vi "Compute Gated Phase Lifetime Plot.vi"(8 "Error In":errorcluster, 9 "Compute Delta Tau":bool, 10 "Phasor Parameters":T1={"Display Parameters"={"# Points"=0, "Ramp Type"=enum."Linear", "Type of Series"=enum."1-Exp Decays", "Min tau"=0.0, "Max tau"=0.0, "Include 0"=FALSE, "Include Infinity"=FALSE}, "Phasor Parameters"={"Harmonic Frequency"=0.0, "Use f* = 1/D Frequency"=FALSE, "Calibrated Phasor"=FALSE, "Calibration Lifetime"=1e-09, "Phasor Calculation"=enum."Direct Sum", "SEPL Type"=enum."UC", "# Gates"=1.0, "Square Gate Width"=1e-09, "Show Ticks"=FALSE}, "Decay & IRF Parameters"={"Lifetime"=0.0, "IRF Offset"=0.0, "IRF Period"=0.0, "Normalized Decays"=FALSE, "IRF Model"=enum."Dirac", "IRF Parameter 1"=0.0}, "Gate Parameters"={"First Gate Start"=0.0, "Use Gate Center"=FALSE, "Gate Width"=0.0, "Gate Step"=0.0, "# Gates"=0.0, "Gate Type"=enum."Square", "Edge Width"=0.0, "Top Slope"=0.0, "Reversed Sawtooth?"=FALSE, "Analytical Computation"=FALSE, "Integration"=enum."Item 0", "Tolerance"=1.0, "# Steps"=1.0, "Type of User-defined Function"=enum."Gate", "Use Gate Step"=FALSE}, "Detector Parameters"={"Frames/Image"=0, "Gates/Frame"=0, "Bits/Frame"=0, "Multiplicity"=0, "Incident Signal"=0.0, "Poisson Signal"=FALSE}} {"Detector Parameters"."Frames/Image" min=1; "Detector Parameters"."Multiplicity" min=0; "Detector Parameters"."Bits/Frame" min=1; "Detector Parameters"."Gates/Frame" min=1; "Gate Parameters"."# Steps" min=0.0; "Gate Parameters"."Tolerance" min=0.0; "Gate Parameters"."Top Slope" min=0.0; "Gate Parameters"."Edge Width" min=0.0; "Gate Parameters"."Gate Step" min=0.0; "Gate Parameters"."# Gates" min=0.0 step=1.0; "Gate Parameters"."Gate Width" min=0.0; "Decay & IRF Parameters"."Lifetime" min=0.0; "Decay & IRF Parameters"."IRF Period" min=0.0; "Phasor Parameters"."Square Gate Width" min=0.0; "Phasor Parameters"."# Gates" min=0.0; "Phasor Parameters"."Calibration Lifetime" min=0.0; "Phasor Parameters"."Harmonic Frequency" min=0.0; "Display Parameters"."Min tau" min=0.0; "Display Parameters"."Max tau" min=0.0; "Display Parameters"."# Points" min=1 step=1}, 11 "P-tau_ph(tau) Graph Refnum":refnum<vi>) -> (0 "Error Out":errorcluster)   [LabVIEW 2019]
uses:
  SEPL Parameters.ctl
  Phasor Explorer Display Parameters.ctl
  Type of Series.ctl
  Phasor Explorer Phasor Parameters.ctl
  Phasor Calculation Type.ctl
  SEPL Type.ctl
  Phasor Explorer Decay Parameters.ctl
  IRF Model.ctl
  Phasor Explorer Gate Parameters.ctl
  Gate Type.ctl
  Type of User-defined Function.ctl
  Phasor Explorer Detector Parameters.ctl
  Phasor L_N[W] Parameters.ctl
  Phasor_Abort Parallel Computation.vi
  <vilib>/Utility/error.llb/Error Cluster From Error Code.vi
  <vilib>/ErrorRing/Error Ring.xnode
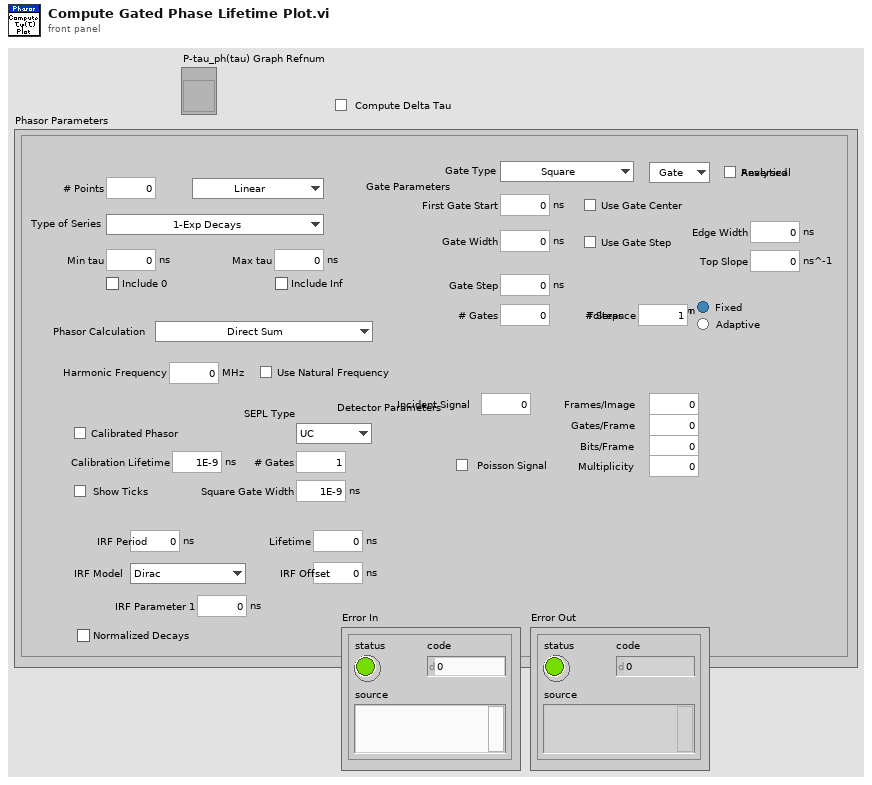
[diagram p1: front panel]
types:
  T1 = typedef "SEPL Parameters.ctl" = cluster{"Display Parameters":T2, "Phasor Parameters":T4, "Decay & IRF Parameters":T7, "Gate Parameters":T9, "Detector Parameters":T12}
  T2 = typedef "Phasor Explorer Display Parameters.ctl" = cluster{"# Points":i32, "Ramp Type":enum16{"Linear", "Logarithmic"}, "Type of Series":T3, "Min tau":dbl[unit], "Max tau":dbl[unit], "Include 0":bool, "Include Infinity":bool}
  T3 = typedef "Type of Series.ctl" = enum16{"1-Exp Decays", "Linear Combination of 1-Exp"}
  T4 = typedef "Phasor Explorer Phasor Parameters.ctl" = cluster{"Harmonic Frequency":dbl[unit], "Use f* = 1/D Frequency":bool, "Calibrated Phasor":bool, "Calibration Lifetime":dbl[unit], "Phasor Calculation":T5, "SEPL Type":T6, "# Gates":dbl, "Square Gate Width":dbl[unit], "Show Ticks":bool}
  T5 = typedef "Phasor Calculation Type.ctl" = enum16{"Direct Sum", "Analytical Formula"}
  T6 = typedef "SEPL Type.ctl" = enum16{"UC", "L_N", "L_N[W]", "L_X"}
  T7 = typedef "Phasor Explorer Decay Parameters.ctl" = cluster{"Lifetime":dbl[unit], "IRF Offset":dbl[unit], "IRF Period":dbl[unit], "Normalized Decays":bool, "IRF Model":T8, "IRF Parameter 1":dbl[unit]}
  T8 = typedef "IRF Model.ctl" = enum16{"Dirac", "Exponential"}
  T9 = typedef "Phasor Explorer Gate Parameters.ctl" = cluster{"First Gate Start":dbl[unit], "Use Gate Center":bool, "Gate Width":dbl[unit], "Gate Step":dbl[unit], "# Gates":dbl, "Gate Type":T10, "Edge Width":dbl[unit], "Top Slope":dbl[unit], "Reversed Sawtooth?":bool, "Analytical Computation":bool, "Integration":enum32{"Item 0", "Item 1"}, "Tolerance":dbl, "# Steps":dbl, "Type of User-defined Function":T11, "Use Gate Step":bool}
  T10 = typedef "Gate Type.ctl" = enum16{"Square", "Finite Edge Square", "Finite Edge, Tilted Top Square", "Triangle", "Sawtooth", "User-defined"}
  T11 = typedef "Type of User-defined Function.ctl" = enum16{"Gate", "IRF"}
  T12 = typedef "Phasor Explorer Detector Parameters.ctl" = cluster{"Frames/Image":i32, "Gates/Frame":i32, "Bits/Frame":i32, "Multiplicity":i32, "Incident Signal":dbl, "Poisson Signal":bool}
  T13 = typedef "Phasor L_N[W] Parameters.ctl" = cluster{"Laser Period":dbl[unit], "Gate Width":dbl[unit], "Gate Step":dbl[unit], "Harmonic frequency":dbl[unit], "IRF offset":dbl[unit], "# Gates":dbl}
  T14 = typedef "Gate Definitions.ctl" = cluster{"First Gate: t1":ext, "Gate Width: W":ext, "Gate Step: d":ext, "# Gates: G":ext, "Use Gate Center":bool, "Frames/Image: F":i32, "Gates/Frame: L":i32, "Bits/Frame: q":i32, "Multiplicity: p":i32, "Gate Type":T10, "Gate Edge s":ext, "Gate Top Slope":ext, "Reversed Sawtooth?":bool, "Computation":bool, "User-defined Gate":T15, "Tolerance":ext, "Integration":enum32{"Item 0", "Item 1"}, "# Steps":ext, "Type of User-defined Function":enum32{"Gate", "IRF"}}
  T15 = typedef "XY Plot Data.ctl" = cluster{"X Array":dbl[], "Y Array":dbl[]}
  T16 = typedef "Decay Definiton.ctl" = cluster{"offset: t0":ext, "period: T":ext, "lifetime: tau":ext, "Incident Signal: I":ext, "Normalized Decays":bool, "IRF Model":T8, "IRF Parameter 1":ext, "Poisson Signal":bool}
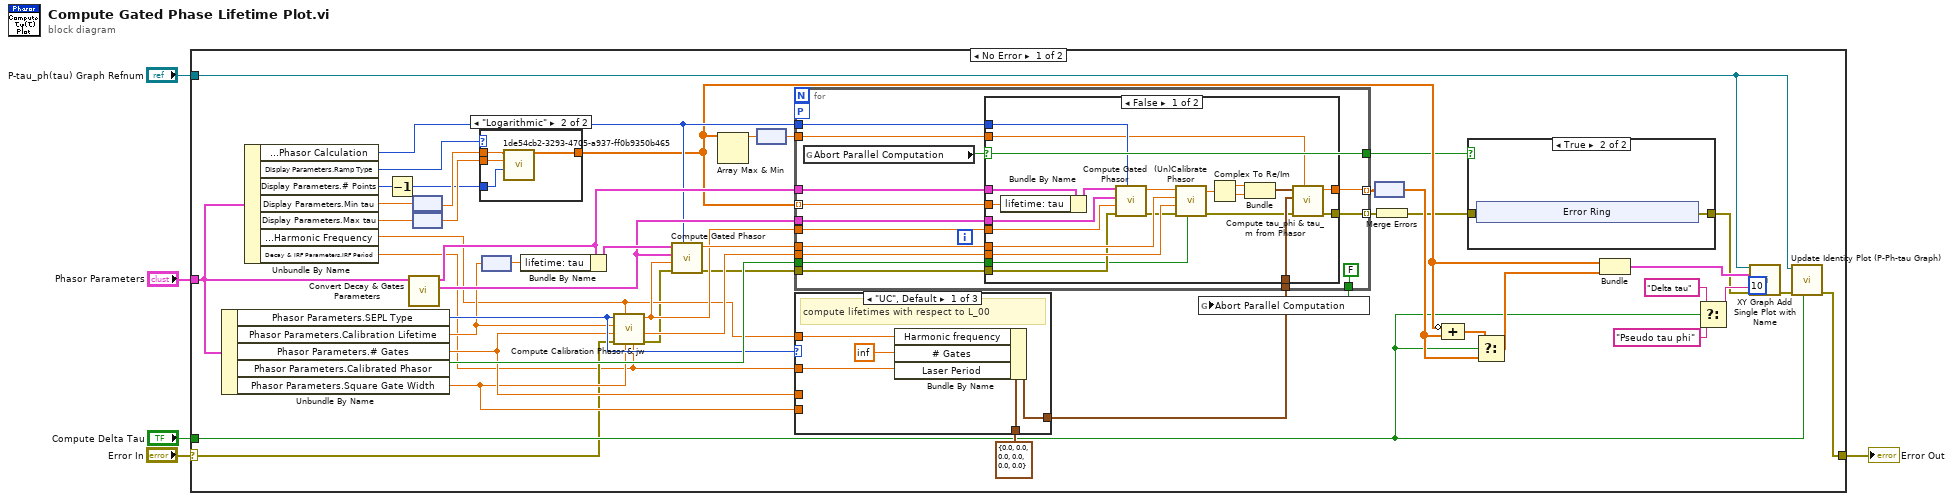
[diagram p0: block diagram]
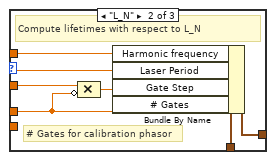
[diagram p3: hidden frame]
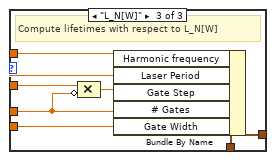
[diagram p4: hidden frame]
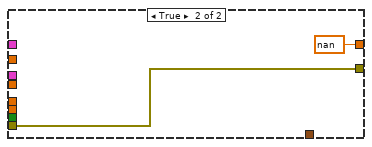
[diagram p5: hidden frame]
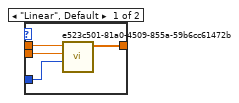
[diagram p6: hidden frame]
diagram:
  n1 = case shown="No Error" "Error In" {
    selector: "Error In" -> [w11 w124]
    tunnel: "Phasor Parameters" -> [w22 _]
    tunnel: "P-tau_ph(tau) Graph Refnum" -> [w41 _]
    tunnel: [w39 w124] -> w2
    tunnel: "Compute Delta Tau" -> [w13 _]
    frame No Error {
      (unwired) 10 ("Max Legend Size (8)")
      n2 = Unbundle By Name(w22) -> ("Phasor Parameters.SEPL Type"=w23:T6, "Phasor Parameters.Calibration Lifetime"=w18:dbl[unit], "Phasor Parameters.# Gates"=w19:dbl, "Phasor Parameters.Calibrated Phasor"=w36:bool, "Phasor Parameters.Square Gate Width"=w16:dbl[unit])
      n3 = Unbundle By Name(w22) -> ("Phasor Parameters.Phasor Calculation"=w35:T5, "Display Parameters.Ramp Type"=w44:enum16{"Linear", "Logarithmic"}, "Display Parameters.# Points"=w43:i32, "Display Parameters.Min tau"=w52:dbl[unit], "Display Parameters.Max tau"=w53:dbl[unit], "Phasor Parameters.Harmonic Frequency"=w17:dbl[unit], "Decay & IRF Parameters.IRF Period"=w6:dbl[unit])
      n4 = Decrement(x=w43) -> (x-1=w42:i32)
      n5 = call "Convert Decay & Gates Parameters.vi"("Phasor Parameters"=w22) -> ("Gates Definitions"=w37:T14, "Decay Definition"=w38:T16)  [unwired: 9 in]
      n6 = node(w52) -> (w46:dbl)
      n7 = node(w53) -> (w47:dbl)
      n8 = case shown="\"Logarithmic\"" w44 {
        tunnel: w47 -> [w119 w121]
        tunnel: w46 -> [w118 w122]
        tunnel: [w117 w120] -> w26
        tunnel: w42 -> [w116 w123]
        frame "Linear", Default {
          n9 = call "e523c501-81a0-4509-855a-59b6cc61472b.vi"("# Steps (1)"=w116, "End (1)"=w119, "Start (0)"=w118) -> ("Ramp"=w117:dbl[])  [unwired: 6 in, 2 out]
        }
        frame "Logarithmic" {
          n10 = call "1de54cb2-3293-4705-a937-ff0b9350b465.vi"("# Steps (1)"=w123, "End (1)"=w121, "Start (1)"=w122) -> ("Ramp"=w120:dbl[])  [unwired: 7 in, 1 out]
        }
      }
      n11 = node(w18) -> (w49:dbl)
      n12 = Bundle By Name(cluster=w38, "lifetime: tau"=w49) -> (w50:T16)
      n13 = call "Compute Calibration Phasor & jw.vi"("Laser Period"=w6, "Gate Width"=w16, "Harmonic frequency"=w17, "Error In"=w11, "# Gates"=w19, "Calibration Lifetime"=w18, "Calibration Phasor Type"=w23) -> ("Error Out"=w10:errorcluster, "z (tau_cal)"=w27:cdb, "i 2 pi f (GHz)"=w28:cdb)  [unwired: 2 in]
      n14 = call "Compute Gated Phasor.vi"("Phasor Calculation Type"=w35, "Error In"=w10, "j 2 pi f"=w28, "Gates Definitions"=w37, "Decay Definition"=w50) -> ("Error Out"=w15:errorcluster, "phasor"=w48:cxt)  [unwired: 4 in, 1 out]
      n15 = Array Max & Min(array=w26) -> (max value=w25:dbl)  [unwired: 3 out]
      n16 = node(w25) -> (w24:dbl[unit])
      n17 = case shown="\"UC\", Default" w23 {
        tunnel: [w64 w70 w77] -> w21
        tunnel: T13 {"Laser Period"=0.0, "Gate Width"=0.0, "Gate Step"=0.0, "Harmonic frequency"=0.0, "IRF offset"=0.0, "# Gates"=0.0} ("Phasor UCN[W] Parameters") -> [w62 w69 w76]
        tunnel: w6 -> [w61 w66 w73]
        tunnel: w17 -> [w60 w68 w75]
        tunnel: w19 -> [_ w67 w74]
        tunnel: w16 -> [_ _ w71]
        frame "UC", Default {
          # "compute lifetimes with respect to L_00"
          n18 = Bundle By Name(cluster=w62, "Harmonic frequency"=w60, "# Gates"=inf ("Gate Parameters.# Gates"), "Laser Period"=w61) -> (w64:T13)
        }
        frame "L_N" {
          # "# Gates for calibration phasor"
          # "Compute lifetimes with respect to L_N"
          n19 = Compound Arithmetic op=MULTIPLY(w66, invert w67) -> (w65:dbl[unit])
          n20 = Bundle By Name(cluster=w69, "Harmonic frequency"=w68, "Laser Period"=w66, "Gate Step"=w65, "# Gates"=w67) -> (w70:T13)
        }
        frame "L_N[W]" {
          # "Compute lifetimes with respect to L_N[W]"
          n21 = Compound Arithmetic op=MULTIPLY(w73, invert w74) -> (w72:dbl[unit])
          n22 = Bundle By Name(cluster=w76, "Harmonic frequency"=w75, "Laser Period"=w73, "Gate Step"=w72, "# Gates"=w74, "Gate Width"=w71) -> (w77:T13)
        }
      }
      n23 = for {
        tunnel: w48 -> [w92]
        tunnel: w27 -> [w91]
        tunnel: w36 -> [w90]
        tunnel: w28 -> [w89]
        tunnel: w37 -> [w86]
        tunnel: w38 -> [w87]
        tunnel: w26 -> [w88] mode=indexing
        tunnel: [w83] -> w45 mode=indexing
        tunnel: w35 -> [w85]
        tunnel: w24 -> [w84]
        tunnel: w21 -> [w82]
        workers-P: _ -> [_]
        tunnel: [FALSE ("Abort")] -> w12
        tunnel: [w78] -> w9
        tunnel: [w80] -> w14 mode=indexing
        tunnel: w15 -> [w79]
        n24 = global read "Phasor_Abort Parallel Computation.vi" "Abort Parallel Computation"() -> (w78:bool)
        n25 = case shown="False" w78 {
          tunnel: w92 -> [w113 _]
          tunnel: w91 -> [w112 _]
          tunnel: w90 -> [w95 _]
          tunnel: w89 -> [w111 _]
          tunnel: w88 -> [w110 _]
          tunnel: w87 -> [w109 _]
          tunnel: w86 -> [w107 _]
          tunnel: w85 -> [w102 _]
          tunnel: w84 -> [w99 _]
          tunnel: [w100 dbl[unit] nan ("tau_ph")] -> w83
          tunnel: w82 -> [w98 _]
          tunnel: [w97 w114] -> w80
          tunnel: w79 -> [w96 w114]
          frame False {
            n26 = Bundle By Name(cluster=w109, "lifetime: tau"=w110) -> (w108:T16)
            n27 = call "Compute Gated Phasor.vi"("Phasor Calculation Type"=w102, "Error In"=w96, "j 2 pi f"=w111, "Gates Definitions"=w107, "Decay Definition"=w108) -> ("Error Out"=w94:errorcluster, "phasor"=w106:cxt)  [unwired: 4 in, 1 out]
            n28 = call "(Un)Calibrate Phasor.vi"("Calibrated Phasor"=w95, "Error In"=w94, "Target Phasor"=w112, "Calibration Phasor"=w113, "Phasor in"=w106) -> ("Error Out"=w93:errorcluster, "Phasor out"=w105:cxt)  [unwired: 5 in]
            n29 = Complex To Re/Im(x + iy=w105) -> (x=w104:ext, y=w103:ext)
            n30 = Bundle(w104, w103) -> (w101:cluster{ext, ext})  [unwired: 1 in]
            n31 = call "Compute tau_phi & tau_m from Phasor.vi"("max tau"=w99, "Error In"=w93, "Phasor L_N[W] Parameters"=w98, "Phasor"=w101) -> ("Error Out"=w97:errorcluster, "tau_ph"=w100:dbl[unit])  [unwired: 5 in, 1 out]
          }
          frame True {
          }
        }
      }
      n32 = global write "Phasor_Abort Parallel Computation.vi" "Abort Parallel Computation"(w12) -> ()
      n33 = node(w45) -> (w33:dbl[])
      n34 = Merge Errors(w14) -> (w8:errorcluster)
      n35 = Compound Arithmetic op=ADD(invert w26, w33) -> (w32:dbl[])
      n36 = case shown="True" w9 {
        tunnel: w8 -> [w54 _]
        tunnel: [w54 w55] -> w7
        frame False {
        }
        frame True {
          n37 = xnode "Error Ring"() -> ("error out"=w55:errorcluster)
        }
      }
      n38 = Select(t=w32, s=w13, f=w33) -> (s? t:f=w34:dbl[])
      n39 = Bundle("Ramp"=w26, w34) -> (w51:cluster{"Ramp":dbl[], dbl[]})  [unwired: 1 in]
      n40 = Select(t="Delta tau" ("Plot Name (\"Plot\")"), s=w13, f="Pseudo tau phi" ("Plot Name (\"Plot\")")) -> (s? t:f=w31:string)
      n41 = call "XY Graph Add Single Plot with Name.vi"("XYGraph Ref in"=w41, "Plot"=w51, "Plot Name (\"Plot\")"=w31, "error in (no error)"=w7) -> ("error out"=w40:errorcluster)  [unwired: 8 in, 3 out]
      n42 = call "Update Identity Plot (P-Ph-tau Graph).vi"("Delta tau"=w13, "error in (no error)"=w40, "XYGraph in"=w41) -> ("error out"=w39:errorcluster)  [unwired: 8 in]
    }
    frame Error {
    }
  }
  "Error Out" <- w2
